vi "globalVarII.vi"() -> ()   [LabVIEW 2020]
panel:
  in  "% of NaN":sgl=60.0
  in  "number of zeros numérique":i32=50
  in  "Counts_Emulate":i64
  in  "BG-level":i32
  in  "Main Path":path
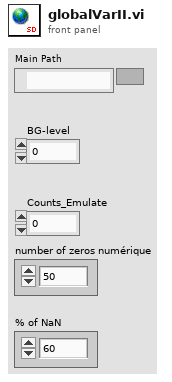
[diagram p1: front panel]
diagram:
